vi "String - Sort Array.vi"(9 "Force Running Numbers":bool, 10 "Check and Add Empty Row if Needed":bool, 11 "2D Array in":string[][](array[string])) -> (1 "Duplicate Index":bool, 2 "Sorted Index":i32[](array[numeric]), 3 "2D Array out":string[][](array[string]))   [LabVIEW 2013]
panel:
  out "sorted array":i32[](array[numeric])
  out "number":i32[](array[numeric])
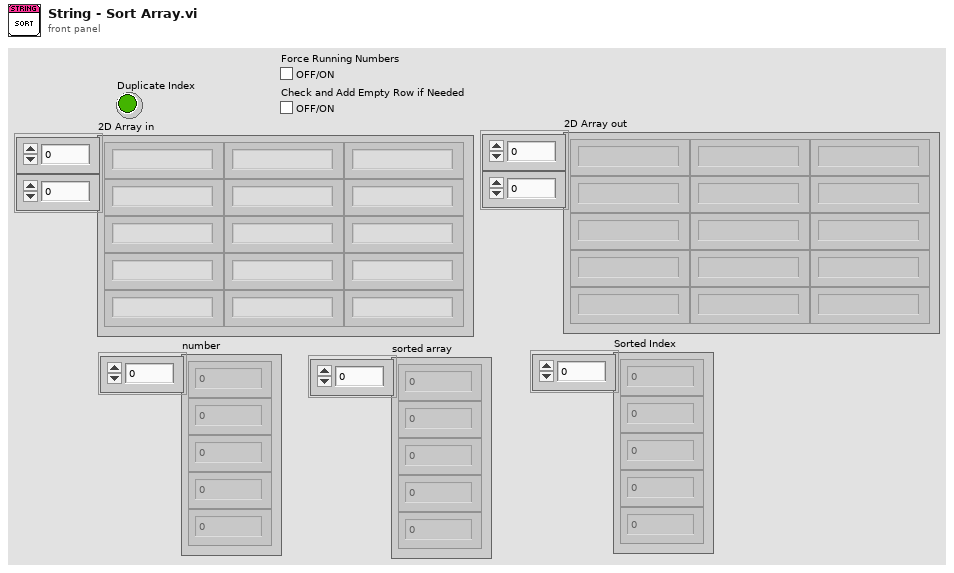
[diagram p1: front panel]
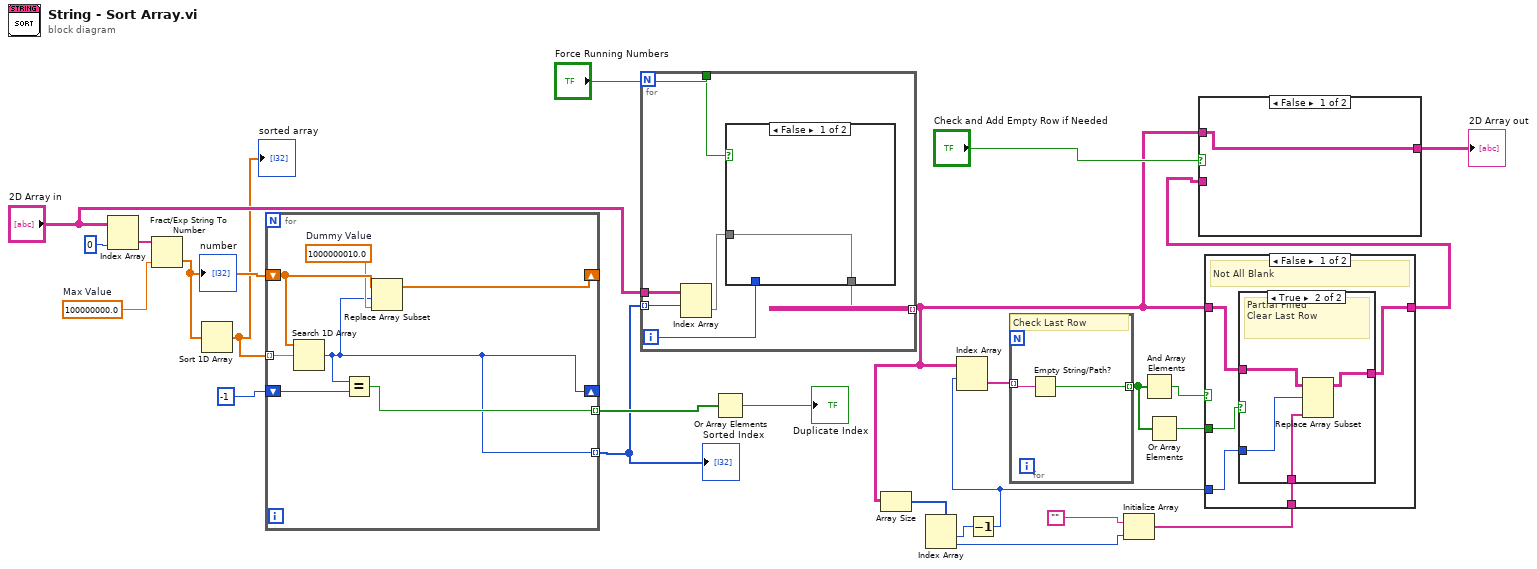
[diagram p0: block diagram]
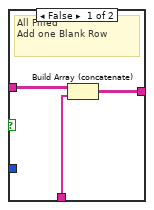
[diagram p3: hidden frame]
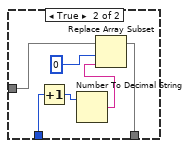
[diagram p5: hidden frame]
diagram:
  w25 = 100000000.0  # Max Value
  n1 = Index Array(array="2D Array in", index (col)=0 ("disabled index (col)")) -> (element=w18:string[])  [unwired: 1 in]
  n2 = Fract/Exp String To Number(string=w18, default (0 dbl)=w25) -> (number=w23:dbl[])  [unwired: 2 in, 1 out]
  "number" <- w23
  n3 = Sort 1D Array(array=w23) -> (sorted array=w19:dbl[])
  "sorted array" <- w19
  n4 = for {
    tunnel: w19 -> [w32] mode=indexing
    shift-right: [w26] -> _
    shift-left: -1 ("index of element") -> [w31]
    tunnel: [w30] -> w21 mode=indexing
    shift-right: [w28] -> _
    shift-left: w23 -> [w29]
    tunnel: [w26] -> w16 mode=indexing
    w27 = 1000000010.0  # Dummy Value
    n5 = Search 1D Array(1D array=w29, element=w32) -> (index of element=w26:i32)  [unwired: 1 in]
    n6 = Equal?(x=w26, y=w31) -> (x = y?=w30:bool)
    n7 = Replace Array Subset(array=w29, new element=w27, index=w26) -> (w28:dbl[])
  }
  "Sorted Index" <- w16
  n8 = for {
    tunnel: "2D Array in" -> [w38]
    tunnel: [w33] -> w2 mode=indexing
    tunnel: w16 -> [w37] mode=indexing
    tunnel: "Force Running Numbers" -> [w36]
    i -> [w34]
    n9 = Index Array(array=w38, index (row)=w37) -> (element=w35:string[])  [unwired: 1 in]
    n10 = case shown="False" w36 {
      tunnel: w35 -> [w39 w45]
      tunnel: w34 -> [_ w43]
      tunnel: [w39 w40] -> w33
      frame False {
      }
      frame True {
        n11 = Increment(x=w43) -> (x+1=w42:i32)
        n12 = Number To Decimal String(number=w42) -> (decimal integer string=w41:string)  [unwired: 1 in]
        n13 = Replace Array Subset(array=w45, new element=w41, index=0) -> (w40:string[])
      }
    }
  }
  n14 = Or Array Elements(Boolean array=w21) -> (logical OR=→"Duplicate Index":bool)
  n15 = Array Size(array=w2) -> (size(s)=w11:i32[])
  n16 = Index Array(array=w11) -> (element #1=w10:i32, element #2=w9:i32)  [unwired: 2 in]
  n17 = Decrement(x=w10) -> (x-1=w6:i32)
  n18 = Index Array(array=w2, index (row)=w6) -> (element=w15:string[])  [unwired: 1 in]
  n19 = for {
    tunnel: w15 -> [w47] mode=indexing
    tunnel: [w46] -> w13 mode=indexing
    # "Check Last Row"
    n20 = Empty String/Path?(string/path=w47) -> (empty?=w46:bool)
  }
  n21 = Initialize Array("", w9) -> (w7:string[])
  n22 = And Array Elements(Boolean array=w13) -> (logical AND=w14:bool)
  n23 = Or Array Elements(Boolean array=w13) -> (logical OR=w12:bool)
  n24 = case shown="False" w14 {
    tunnel: w2 -> [w51 w60]
    tunnel: [w49 w60] -> w4
    tunnel: w12 -> [w52 _]
    tunnel: w7 -> [w50 _]
    tunnel: w6 -> [w48 _]
    frame False {
      # "Not All Blank"
      n25 = case shown="True" w52 {
        tunnel: w51 -> [w55 w59]
        tunnel: w50 -> [w54 w57]
        tunnel: [w53 w56] -> w49
        tunnel: w48 -> [_ w58]
        frame False {
          # "All Filled\nAdd one Blank Row"
          n26 = Build Array (concatenate)(w55, w54) -> (w53:string[][])
        }
        frame True {
          # "Partial Filled\nClear Last Row"
          n27 = Replace Array Subset(array=w59, new element=w57, index (row)=w58) -> (w56:string[][])  [unwired: 1 in]
        }
      }
    }
    frame True {
      # "Last Row All Blank"
    }
  }
  n28 = case shown="False" "Check and Add Empty Row if Needed" {
    tunnel: w4 -> [_ w62]
    tunnel: [w61 w62] -> w3
    tunnel: w2 -> [w61 _]
    frame False {
    }
    frame True {
    }
  }
  "2D Array out" <- w3
